vi "ULx Acq&Graph Voltage-Int Clk.vi"() -> ()   [LabVIEW 2016]
doc: "I. Description:\nThis example demonstrates how to acquire a finite amount of data (waveform) using the DAQ device's internal clock.\n\nII. Instructions for Running:\n1. Select the physical channel to correspond to where your signal is input on the DAQ device.\n2. Enter the minimum and maximum voltages.\nNote: For better accuracy try to match the input range to the expected voltage level of the measured signal.\n3. Select the number of samples to acquire.\n4. Set the rate of the acquisition\nNote: The rate should be AT LEAST twice as fast as the maximum frequency component of the signal being acquired.\n\nIII. Block Diagram Steps:\n1. Create an analog input voltage channel.\n2. Set the rate for the sample clock. Additionally, define the sample mode to be finite and set the number of samples to be acquired per channel.\n3. Call the Start VI to start the acquisition.\n4. Use the Read VI to measure multiple samples from N Channels on the device. Set a timeout so an error is returned if the samples are not returned in the specified time limit\n5. Call the Clear Task VI to clear the Task.\n6. Use the popup dialog box to display an error if any.\n \nIV. I/O Connections Overview:\nMake sure your signal input terminal matches the Physical Channel I/O Control. For further connection information, refer to your hardware reference manual."
uses:
  <vilib>/Utility/error.llb/DialogType.ctl
  <vilib>/ULx/Create Channel.llb/ULx Create Channel (AI-Voltage-Basic).vi
  <vilib>/ULx/Timing.llb/ULx Timing (Sample Clock).vi
  <vilib>/ULx/Read.llb/ULx Read (Analog 1D Wfm NChan NSamp).vi
  <vilib>/measure/madcrms.llb/Basic Averaged DC-RMS for 1 Chan.vi
  <vilib>/measure/NI_MAPro.lvlib
panel:
  in  "error in (no error)":errorcluster
  out "error out":errorcluster
  in  "Window Size":i32
  in  "Window Data":bool
  out "XY Graph":cluster{"Y":dbl[], "Y":dbl[]}[](graph)
  out "Time (s)":dbl
  out "loop":i32
  in  "stop":bool
  out "In Range?":bool
  out "Elapsed ms":u32
  in  "Channel Data Rate S/s":dbl=3720.0 format="%#_13g"
  out "Number of Channels":u16
  out "Acq Time (s)":dbl
  out "timeout":dbl=10.0 format="%0.2f"
  in  "Physical Channel":refnum<k21>="Dev0/Ai8"
  in  "Maximum Value":dbl=10.0 format="%0.2f"
  in  "Minimum Value":dbl=-10.0 format="%0.2f"
  out "Rate":dbl=1000.0 caption="Sample Rate (Hz)"
  in  "Samples per Channel":i32=1000
  out "Measurement":waveform(dbl)[](graph)
  # "For instructions, select Help>>Show Context Help"
  # "Channel Parameters"
  # "Timing Parameters"
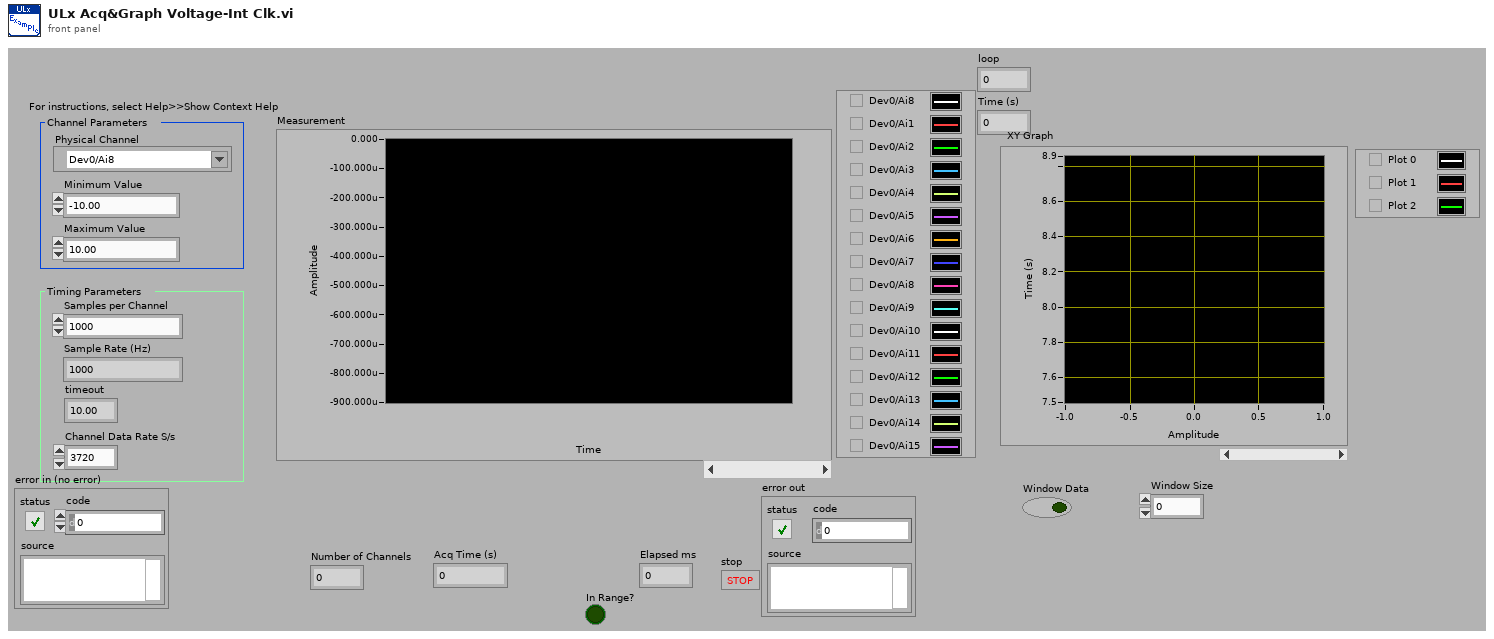
[diagram p1: front panel]
types:
  T1 = typedef "DialogType.ctl" = u16
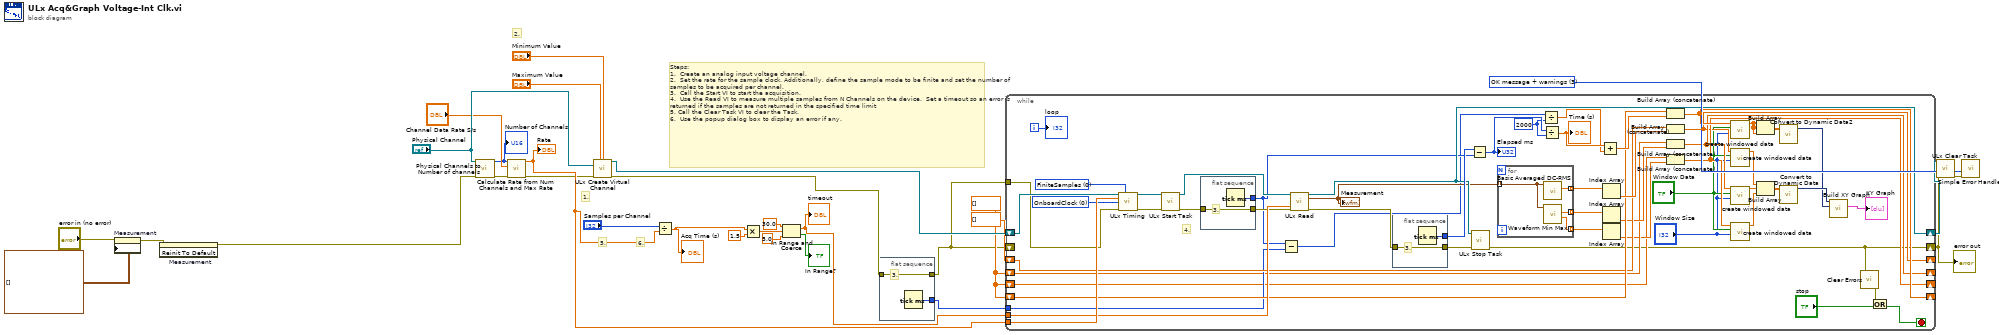
[diagram p0: block diagram]
diagram:
  w3 = dbl[] []
  w29 = T1 3 items=["no dialog", "OK message", "continue or stop message", "OK message + warnings", "continue/stop + warnings"] ("type of dialog (OK msg:1)")
  # "6."
  # "5."
  # "Steps: \n1.  Create an analog input voltage channel.\n2.  Set the rate for the sample clock. Additionally, define the sample mode to be finite and set the number of samples to be acquired per channel.\n3.  Call the Start VI to start the acquisition.\n4.  Use the Read VI to measure multiple samples from N Channels on the device.  Set a timeout so an error is returned if the samples are not returned in the specified time limit\n5. Call the Clear Task VI to clear the Task.\n6.  Use the popup dialog box to display an error if any."
  # "2."
  # "1."
  n1 = property on="Measurement" class="WFChart (strict)"(error in="error in (no error)", "History Data"=waveform(dbl)[][] []) -> (error out=w8:errorcluster)  [unwired: 1 in, 1 out]
  n2 = invoke on="Measurement" class="WFChart (strict)" method="Reinit To Default"(error in=w8) -> (error out=w11:errorcluster)  [unwired: 2 in, 2 out]
  n3 = call "Physical Channels to Number of channels.vi"("error in (no error)"=w11, "Physical Channel in"="Physical Channel") -> ("error out"=w10:errorcluster, "Number of Channels"=w23:i32)  [unwired: 7 in, 1 out]
  "Number of Channels" <- w23
  n4 = call "Calculate Rate from Num Channels and Max Rate.vi"("error in (no error)"=w10, "Channel Data Rate S/s"="Channel Data Rate S/s", "Number of Channels"=w23) -> ("error out"=w9:errorcluster, "Rate"=w22:dbl)  [unwired: 7 in]
  "Rate" <- w22
  n5 = call-poly <vilib>:"ULx Create Virtual Channel.vi"("maximum value"="Maximum Value", "minimum value"="Minimum Value", "physical channels"="Physical Channel", "error in"=w9) -> ("task out"=w30:refnum<k24>, "error out"=w5:errorcluster)  [unwired: 10 in]
  n6 = Divide(x="Samples per Channel", y=w22) -> (x/y=w21:dbl)
  "Acq Time (s)" <- w21
  n7 = Multiply(x=w21, y=1.5) -> (x*y=w19:dbl)
  n8 = In Range and Coerce(upper limit=30.0, x=w19, lower limit=5.0) -> (coerced(x)=w16:dbl, In Range?=→"In Range?":bool)
  "timeout" <- w16
  n9 = flat-sequence {
    tunnel: [w32] -> w1
    tunnel: w5 -> [w32]
    tunnel: [w31] -> w4
    frame #0 {
      # "3."
      n10 = Tick Count (ms)() -> (millisecond timer value=w31:u32)
    }
  }
  n11 = while {
    tunnel: w22 -> [w84]
    tunnel: w16 -> [w83]
    shift-right: [w35] -> w13
    shift-left: w1 -> [_]
    shift-right: [w72] -> w14
    shift-left: w30 -> [w86]
    shift-right: [w45] -> _
    shift-left: w3 -> [w60]
    shift-right: [w40] -> _
    shift-left: dbl[] [] -> [w59]
    tunnel: w4 -> [w57]
    shift-right: [w42] -> _
    shift-left: w3 -> [w54]
    shift-right: [w44] -> _
    shift-left: w3 -> [w51]
    tunnel: w1 -> [w33]
    i -> [w69]
    stop <- w36 stop-if-true
    w63 = u32 2000 ("y")
    w74 = 0 items=["OnboardClock", "ExternalClock", "NoClock"] ("clock source")
    w75 = 0 items=["FiniteSamples", "ContinuousSamples"] ("sample mode")
    # "4."
    n12 = call-poly <vilib>:"ULx Timing.vi"("task in"=w86, "sample mode"=w75, "rate"=w84, "clock source"=w74, "error in"=w33) -> ("task out"=w85:refnum<k24>, "error out"=w80:errorcluster)  [unwired: 9 in]
    n13 = call <vilib>:"ULx Start Task.vi"("task in"=w85, "error in"=w80) -> ("task out"=w81:refnum<k24>, "error out"=w82:errorcluster)  [unwired: 12 in]
    n14 = flat-sequence {
      tunnel: [w92] -> w77
      tunnel: w82 -> [w92]
      tunnel: [w91] -> w64
      frame #0 {
        # "3."
        n15 = Tick Count (ms)() -> (millisecond timer value=w91:u32)
      }
    }
    n16 = Subtract(x=w64, y=w57) -> (x-y=w58:u32)
    n17 = call-poly <vilib>:"ULx Read.vi"("task in"=w81, "timeout"=w83, "error in"=w77) -> ("task out"=w72:refnum<k24>, "data"=w71:waveform(dbl)[], "error out"=w79:errorcluster)  [unwired: 10 in]
    "Measurement" <- w71
    n18 = flat-sequence {
      tunnel: [w94] -> w73
      tunnel: w79 -> [w94]
      tunnel: [w93] -> w78
      frame #0 {
        # "3."
        n19 = Tick Count (ms)() -> (millisecond timer value=w93:u32)
      }
    }
    n20 = Subtract(x=w78, y=w64) -> (x-y=w70:u32)
    "Elapsed ms" <- w70
    n21 = call <vilib>:"ULx Stop Task.vi"("error in"=w73, "task in"=w72) -> ("error out"=w35:errorcluster)  [unwired: 8 in, 1 out]
    n22 = for {
      tunnel: w71 -> [w89] mode=indexing
      tunnel: [w90] -> w67 mode=indexing
      tunnel: [w88] -> w55 mode=indexing
      tunnel: [w87] -> w53 mode=indexing
      n23 = call-poly <vilib>:"Basic Averaged DC-RMS.vi"("signal in"=w89) -> ("RMS value"=w90:dbl)  [unwired: 7 in, 3 out]
      n24 = call <vilib>:"Waveform Min Max.vi"("waveform in"=w89) -> ("Y min"=w87:dbl, "Y max"=w88:dbl)  [unwired: 5 in, 4 out]
    }
    n25 = Divide(x=w58, y=w63) -> (x/y=w65:dbl)
    n26 = Divide(x=w70, y=w63) -> (x/y=w68:dbl)
    "Time (s)" <- w68
    n27 = Add(x=w68, y=w65) -> (x+y=w66:dbl)
    n28 = Index Array(array=w67) -> (element=w62:dbl)  [unwired: 1 in]
    n29 = Index Array(array=w55) -> (element=w56:dbl)  [unwired: 1 in]
    n30 = Index Array(array=w53) -> (element=w52:dbl)  [unwired: 1 in]
    n31 = Build Array (concatenate)(w60, w66) -> (w45:dbl[])
    n32 = Build Array (concatenate)(w59, w62) -> (w40:dbl[])
    n33 = Build Array (concatenate)(w54, w56) -> (w42:dbl[])
    n34 = Build Array (concatenate)(w51, w52) -> (w44:dbl[])
    n35 = call "create windowed data.vi"("Window Size"="Window Size", "Window Data"="Window Data", "Array in"=w45) -> ("Array out"=w46:dbl[])  [unwired: 8 in]
    n36 = call "create windowed data.vi"("Window Size"="Window Size", "Window Data"="Window Data", "Array in"=w40) -> ("Array out"=w39:dbl[])  [unwired: 8 in]
    n37 = call "create windowed data.vi"("Window Size"="Window Size", "Window Data"="Window Data", "Array in"=w42) -> ("Array out"=w41:dbl[])  [unwired: 8 in]
    n38 = call "create windowed data.vi"("Window Size"="Window Size", "Window Data"="Window Data", "Array in"=w44) -> ("Array out"=w43:dbl[])  [unwired: 8 in]
    n39 = Build Array(w46, w46, w46) -> (w48:dbl[][])
    n40 = Build Array(w39, w41, w43) -> (w50:dbl[][])
    n41 = call "Convert to Dynamic Data2"("2D Array"=w48) -> ("Dynamic Data Type"=w47:dynamicdata)  [unwired: 3 in]
    n42 = call "Convert to Dynamic Data"("2D Array"=w50) -> ("Dynamic Data Type"=w49:dynamicdata)  [unwired: 3 in]
    n43 = call "Build XY Graph"("Y Input"=w47, "X Input"=w49) -> ("XY Graph"=→"XY Graph":cluster{"X":dbl[], "Y":dbl[]}[])  [unwired: 8 in, 1 out]
    n44 = call <vilib>:"Clear Errors.vi"("error in (no error)"=w35) -> ("error out"=w34:errorcluster)  [unwired: 5 in, 1 out]
    n45 = Or(x=w34, y="stop") -> (x .or. y?=w36:bool)
    "loop" <- w69
  }
  "error out" <- w13
  n46 = call <vilib>:"ULx Clear Task.vi"("task in"=w14, "error in"=w13) -> ("error out"=w12:errorcluster)  [unwired: 13 in]
  n47 = call <vilib>:"Simple Error Handler.vi"("type of dialog (OK msg:1)"=w29, "error in (no error)"=w12) -> ()  [unwired: 3 in, 5 out]
